vi "SRDG535.evt Call Set Output.vi"(0 "i ref in":refnum<vi>, 1 "Generator Instance":string="N/A", 2 "Output":T2 items=["T0", "A", "B", "AB", "C", "D", "CD"], 3 "Channel Settings":T1={"Inversion"=FALSE, "Amplitude (V)"=1.0, "Offset (V)"=0.0, "Mode"=0, "Load"=FALSE} {"Mode" items=["TTL", "NIM", "ECL", "VAR"]; "Offset (V)" min=-3.0 max=4.0 format="%.2f"; "Amplitude (V)" min=-3.0 max=4.0 format="%.2f"}, 5 "error IO":errorcluster) -> (14 "i ref out":refnum<vi>, 19 "error out":errorcluster)   [LabVIEW 2014, in "SRDG535.lvlib"]
doc: "This VI sends a simple event call."
uses:
  SRDG535.lvlib
  SRDG535.Channel.ctl
  SRDG535.Channel Output.ctl
  CS_Core/CSSystem/CoreLib/CoreLib.short 2 byte array.vi
  CS_Core/CSSystem/CoreLib/CoreLib.double 2 byte array.vi
  CS_Core/CSSystem/CoreLib/CoreLib.int 2 byte array.vi
  CS_Core/CSSystem/CoreLib/CoreLib.lvlib
  CS_Core/BaseProcess/BaseProcess.lvlib
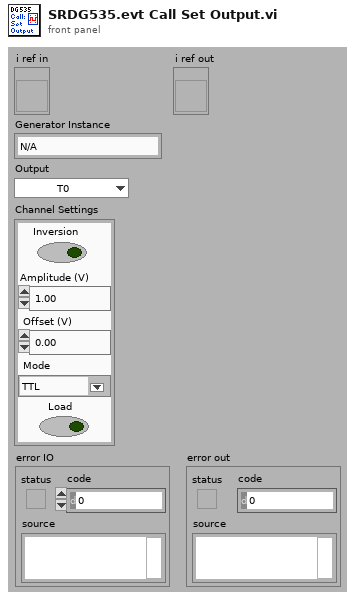
[diagram p1: front panel]
types:
  T1 = typedef "SRDG535.lvlib/SRDG535.Channel Output.ctl" = cluster{"Inversion":bool, "Amplitude (V)":dbl, "Offset (V)":dbl, "Mode":i32, "Load":bool}
  T2 = typedef "SRDG535.lvlib/SRDG535.Channel.ctl" = u16
  T3 = typedef "CoreDefs.rawDataType.ctl" = i8[]
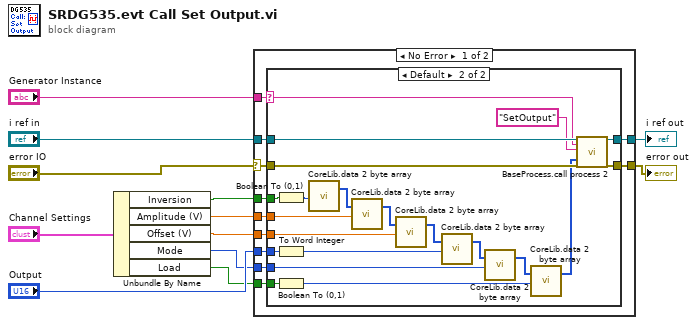
[diagram p0: block diagram]
diagram:
  n1 = Unbundle By Name("Channel Settings") -> ("Inversion"=w5:bool, "Amplitude (V)"=w4:dbl, "Offset (V)"=w3:dbl, "Mode"=w2:i32, "Load"=w1:bool)
  n2 = case shown="No Error" "error IO" {
    selector: "error IO" -> [w23 w47]
    tunnel: "Generator Instance" -> [w13 _]
    tunnel: [w22 w47] -> w12
    tunnel: [w20 w48] -> w11
    tunnel: w1 -> [w14 _]
    tunnel: w2 -> [w15 _]
    tunnel: "Output" -> [w16 _]
    tunnel: w3 -> [w17 _]
    tunnel: w4 -> [w18 _]
    tunnel: w5 -> [w19 _]
    tunnel: "i ref in" -> [w21 w48]
    frame No Error {
      n3 = case shown="Default" w13 {
        selector: w13 -> [_ w34]
        tunnel: w23 -> [w24 w46]
        tunnel: [w24 w45] -> w22
        tunnel: w21 -> [w25 w44]
        tunnel: [w25 w43] -> w20
        tunnel: w19 -> [_ w32]
        tunnel: w18 -> [_ w33]
        tunnel: w17 -> [_ w30]
        tunnel: w16 -> [_ w37]
        tunnel: w15 -> [_ w29]
        tunnel: w14 -> [_ w28]
        frame "", "N/A" {
        }
        frame Default {
          n4 = Boolean To (0,1)(Boolean=w32) -> (0, 1=w31:i16)
          n5 = To Word Integer(number=w37) -> (16bit integer=w36:i16)
          n6 = Boolean To (0,1)(Boolean=w28) -> (0, 1=w27:i16)
          n7 = call-poly "CoreLib.data 2 byte array.vi"("i16"=w31) -> ("byteArray out"=w40:T3)  [unwired: 18 in]
          n8 = call-poly "CoreLib.data 2 byte array.vi"("byteArray"=w40, "f64"=w33) -> ("byteArray out"=w39:T3)  [unwired: 17 in]
          n9 = call-poly "CoreLib.data 2 byte array.vi"("byteArray"=w39, "f64"=w30) -> ("byteArray out"=w38:T3)  [unwired: 17 in]
          n10 = call-poly "CoreLib.data 2 byte array.vi"("byteArray"=w38, "i16"=w36) -> ("byteArray out"=w35:T3)  [unwired: 17 in]
          n11 = call-poly "CoreLib.data 2 byte array.vi"("byteArray"=w35, "i32"=w29) -> ("byteArray out"=w41:T3)  [unwired: 17 in]
          n12 = call-poly "CoreLib.data 2 byte array.vi"("byteArray"=w41, "i16"=w27) -> ("byteArray out"=w26:T3)  [unwired: 17 in]
          n13 = call "BaseProcess.call process 2.vi"("i ref in"=w44, "Object"=w34, "Selector"="SetOutput", "Data"=w26, "error in (no error)"=w46) -> ("i ref out"=w43:refnum<vi>, "error out"=w45:errorcluster)  [unwired: 13 in]
        }
      }
    }
    frame Error {
    }
  }
  "error out" <- w12
  "i ref out" <- w11
